vi "Construct.vi"   [LabVIEW 2019, in "TSC Event Logger.lvlib" / "Text File.lvclass"]
uses:
  Text File.lvclass
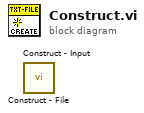
[diagram p0: block diagram]
diagram:
  n1 = call "Construct - Input.vi"() -> ()  [unwired: 10 in, 2 out]
  n2 = call "Construct - File.vi"() -> ()  [unwired: 10 in, 2 out]
